vi "SR785 get display data.vi"(5 "average num":i32=1, 6 "Delay Time (s)":dbl=1.0, 7 "Display (0: Display A)":i32(ring) items=["Display A", "Display B"], 8 "error in (no error)":errorcluster, 11 "VISA resource name":refnum<visa-resource-name>) -> (0 "error out":errorcluster, 3 "Waveform Graph":dbl[](graph))   [LabVIEW 2023]
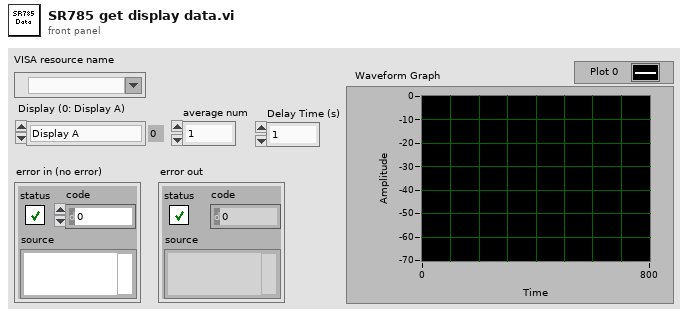
[diagram p1: front panel]
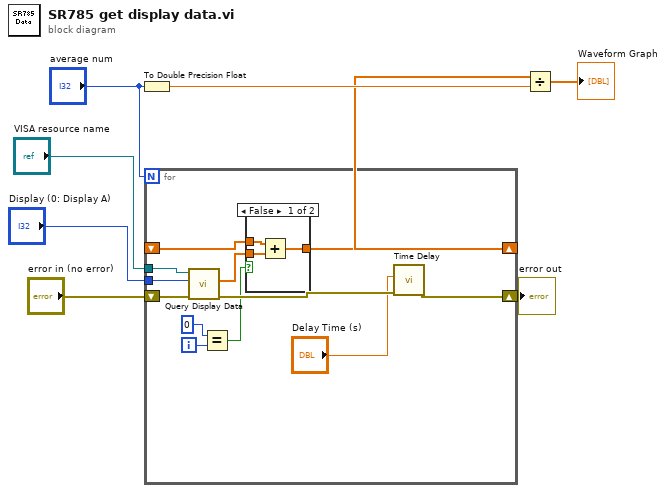
[diagram p0: block diagram]
diagram:
  n1 = To Double Precision Float(number="average num") -> (double precision float=w3:dbl)
  n2 = for {
    N: "average num" -> [_]
    tunnel: "VISA resource name" -> [w18]
    tunnel: "Display (0: Display A)" -> [w17]
    shift-right: [w10] -> w7
    shift-left: "error in (no error)" -> [w20]
    shift-right: [w11] -> w2
    shift-left: _ -> [w12]
    i -> [w16]
    n3 = call <instrlib>:"Query Display Data.vi"("error in (no error)"=w20, "Display (0: Display A)"=w17, "VISA resource name"=w18) -> ("error out"=w19:errorcluster, "Display Data"=w13:dbl[])  [unwired: 6 in, 1 out]
    n4 = Equal?(x=0, y=w16) -> (x = y?=w14:bool)
    n5 = case shown="False" w14 {
      tunnel: w13 -> [w23 w24]
      tunnel: w12 -> [w22 _]
      tunnel: [w21 w24] -> w11
      frame False {
        n6 = Add(x=w22, y=w23) -> (x+y=w21:dbl[])
      }
      frame True {
      }
    }
    n7 = call "Time Delay"("error in (no error)"=w19, "Delay Time (s)"="Delay Time (s)") -> ("error out"=w10:errorcluster)  [unwired: 9 in]
  }
  "error out" <- w7
  n8 = Divide(x=w2, y=w3) -> (x/y=→"Waveform Graph":dbl[])
